vi "MQTT-publisher.vi"() -> ()   [LabVIEW 2020]
uses:
  <vilib>/numeric/Random Number (Range) I64.vi
  <vilib>/numeric/sub_Random U32.vi
  <vilib>/LabVIEW Open Source Project/Connection/Connection.TCP/Connection.TCP.lvclass
  C:/Program Files (x86)/National Instruments/LabVIEW 2020/vi.lib/LabVIEW Open Source Project/Connection/Connection/Connection.lvclass
  <vilib>/LabVIEW Open Source Project/MQTT Client/Client class/Client.lvclass
  C:/Program Files (x86)/National Instruments/LabVIEW 2020/vi.lib/LabVIEW Open Source Project/MQTT Connection/MQTT_Base/Base Class/MQTT_Base.lvclass
  <vilib>/LabVIEW Open Source Project/MQTT Connection/MQTT_Base/Base Class/MQTT_Base.lvclass
panel:
  out "Gauge":dbl(knob) scale=0.0..100.0
  out "Numeric":dbl
  in  "stop":bool
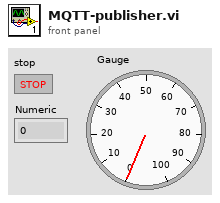
[diagram p1: front panel]
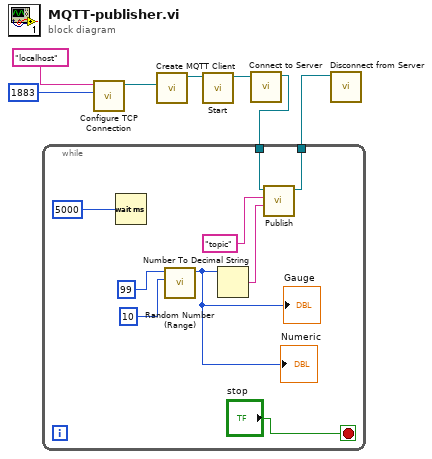
[diagram p0: block diagram]
diagram:
  n1 = call <vilib>:"Configure TCP Connection.vi"("remote port (80)"=1883, "address (localhost)"="localhost") -> ("Connection.TCP"=w7:refnum<class "Connection.TCP.lvclass">)  [unwired: 8 in, 1 out]
  n2 = call <vilib>:"Create MQTT Client.vi"("Connection Configuration"=w7) -> ("Client out"=w4:refnum<class "Client.lvclass">)  [unwired: 9 in, 1 out]
  n3 = call <vilib>:"Start.vi"("MQTT_Base in"=w4) -> ("MQTT_Base out"=w3:refnum<class "Client.lvclass">)  [unwired: 8 in, 2 out]
  n4 = call <vilib>:"Connect to Server.vi"("Client in"=w3) -> ("Client out"=w2:refnum<class "Client.lvclass">)  [unwired: 7 in, 3 out]
  n5 = while {
    tunnel: w2 -> [w10]
    tunnel: [w9] -> w1
    stop <- "stop" stop-if-true
    n6 = Wait (ms)(milliseconds to wait=5000) -> ()  [unwired: 1 out]
    n7 = call-poly <vilib>:"Random Number (Range).vi"("lower bound (-100)"=10, "upper bound (100)"=99) -> ("number"=w12:i64)  [unwired: 9 in]
    "Numeric" <- w12
    "Gauge" <- w12
    n8 = Number To Decimal String(number=w12) -> (decimal integer string=w14:string)  [unwired: 1 in]
    n9 = call <vilib>:"Publish.vi"("Payload"=w14, "Topic Name (empty: Payload name)"="topic", "Client in"=w10) -> ("Client out"=w9:refnum<class "Client.lvclass">)  [unwired: 6 in, 2 out]
  }
  n10 = call <vilib>:"Disconnect from Server.vi"("Client in"=w1) -> ()  [unwired: 8 in, 3 out]
